vi "Send Command.vi"(8 "error in":errorcluster, 9 "Value":variant, 10 "Command":string, 11 "Multimeter in":refnum<class "Multimeter.lvclass">) -> (0 "error out":errorcluster, 3 "Multimeter out":refnum<class "Multimeter.lvclass">)   [LabVIEW 2019, in "Multimeter.lvlib" / "Multimeter.lvclass"]
uses:
  Library/Multimeter.lvclass
  builds/Instruments/Instruments.lvlibp/Library/Instruments.lvclass
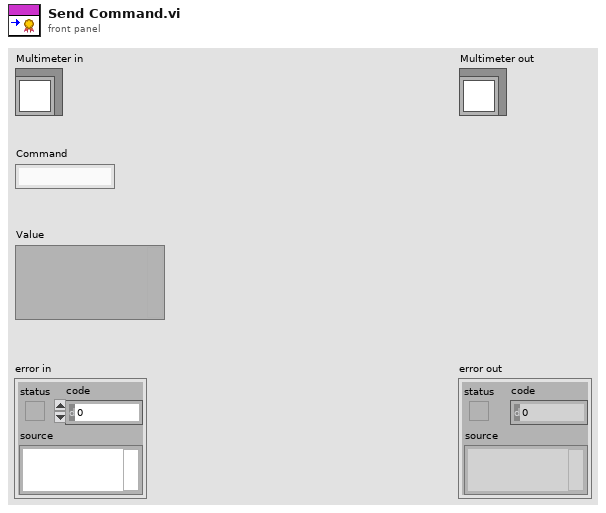
[diagram p1: front panel]
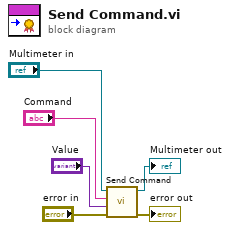
[diagram p0: block diagram]
diagram:
  n1 = call-parent "Send Command.vi"("error in"="error in", "Value"="Value", "Command"="Command", "Instruments in"="Multimeter in") -> ("error out"=→"error out":errorcluster, "Instruments out"=→"Multimeter out":refnum<class "Multimeter.lvclass">)  [unwired: 6 in]
